vi "Main.vi"() -> ()   [LabVIEW 2020]
uses:
  controls/message cluster.ctl
  <vilib>/Platform/TimedLoop/XDataNode/timing_clust.ctl
  <vilib>/Platform/TimedLoop/XDataNode/nitl_modes.ctl
  <vilib>/Platform/TimedLoop/XDataNode/wakeup.ctl
  <instrlib>/Marlin Instrument Driver/Public/controls/move parameters.ctl
  <instrlib>/Marlin Instrument Driver/Public/controls/axes.ctl
  <instrlib>/Marlin Instrument Driver/Public/controls/heater.ctl
  <vilib>/Utility/config.llb/Read Key (String).vi
  <vilib>/Utility/config.llb/Read Key (Double).vi
  <vilib>/Utility/config.llb/Write Key (String).vi
  <vilib>/Utility/config.llb/Write Key (Double).vi
  <vilib>/platform/TimedLoop/XDataNode/XDataNode.xnode
  <instrlib>/Marlin Instrument Driver/Marlin Instrument Driver.lvlib
  <vilib>/Utility/config.llb/NI_LVConfig.lvlib
  <vilib>/Platform/TimedLoop/XDataNode/XDNodeRunTimeDep.lvlib
panel:
  in  "Tab Control":T1(tab)
  in  "Disable steppers":bool
  in  "Chamber temp":enum16{"0", "40", "50", "60", "70", "80"}(ring) caption="Enum"
  in  "Bed temp":enum16{"0", "50", "60", "80", "100", "120"}(ring) caption="Enum"
  in  "Nozzle temp":T2(ring) caption="Enum"
  in  "Speed":u32=1000 caption="mm/min"
  in  "Distance":enum16{"0.1", "1", "10", "100"}(ring)=enum."10" caption="mm"
  in  "Fan control":u8(slide) caption="%" scale=0.0..255.0
  in  "Extrude":bool
  in  "Retract":bool
  in  "Home all":bool caption="ALL"
  in  "Home Z":bool
  in  "Z-":bool
  in  "Z+":bool
  in  "Home XY":bool
  in  "XY-":bool
  in  "X-":bool
  in  "XY+":bool
  in  "X-Y+":bool
  in  "Y-":bool
  in  "X+Y-":bool
  in  "X+":bool
  in  "Y+":bool
  in  "Monitor data":bool caption="Monitoring slows down communication"
  in  "Update frequency":u32=1000 caption="ms"
  out "Temperature Chart":dbl[][](graph)
  out "Z min":bool
  out "Y min":bool
  out "X min":bool
  out "Gcode array":string[](array[string])
  in  "Stop Gcode":bool
  in  "Pause Gcode":bool
  in  "Test mode":bool
  out "XY Graph":cluster{"X":dbl, "Y":dbl}[](graph)
  in  "Start Gcode":bool
  in  "Gcode file":path caption="Path"
  out "Position sent":dbl caption="Numeric"
  in  "Test mode":bool
  in  "Start torture":bool
  in  "Axle":enum16{"X", "Y", "Z"}(ring) caption="Enum"
  in  "Speed":u32(slide)=3000 caption="%" scale=0.0..9000.0
  in  "Distance":dbl(slide)=100.0 caption="%" scale=0.0..300.0
  out "Initialized":bool
  in  "Initialize":bool
  in  "Delete":bool
  in  "Save":bool
  in  "Z":dbl caption="Numeric"
  in  "Y":dbl caption="Numeric"
  in  "X":dbl caption="Build volume"
  in  "COM port":refnum<visa-resource-name>
  in  "3D printer":string(combo) caption="Combo Box"
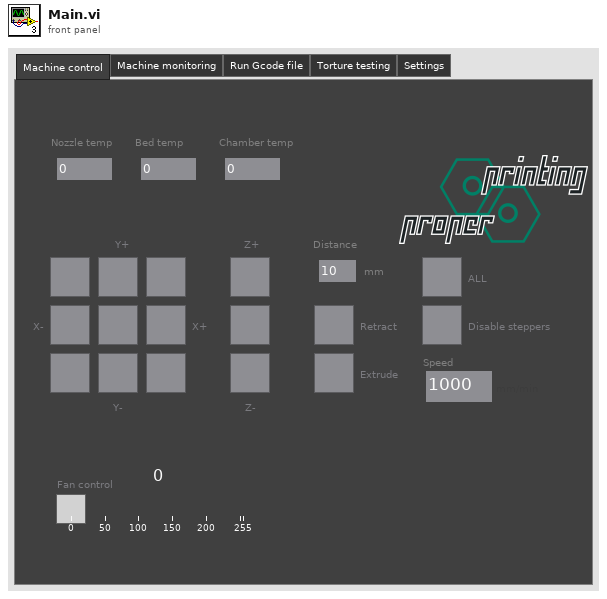
[diagram p1: front panel]
types:
  T1 = enum32{"Machine control", "Machine monitoring", "Run Gcode file", "Torture testing", "Settings"}
  T2 = enum16{"0", "100", "200", "230", "240", "260", "280", "290"}
  T3 = enum8{"Enabled", "Disabled", "Disabled and Grayed Out"}
  T4 = typedef "message cluster.ctl" = cluster{"message":string, "data":variant}
  T5 = typedef "XDNodeRunTimeDep.lvlib/timing_clust.ctl" = cluster{"Expected End [f-1]":u64, "Actual End [f-1]":u64, "Finished Late? [f-1]":bool, "Expected End [i-1]":u64, "Actual End [i-1]":u64, "Finished Late? [i-1]":bool, "Expected Start [i]":u64, "Actual Start [i]":u64, "Expected Start [f]":u64, "Actual Start [f]":u64, "Source Name":string, "Structure Name":string, "Period":i64, "Deadline":i64, "Offset":i64, "Start":i64, "Priority":i32, "Timeout":i32, "Mode":T6, "Wakeup Reason":T7, "Error":errorcluster, "Source Type":string, "Secondary Source Type":string, "Global End Time":u64, "Global Start Time":u64, "Frame Duration":u64, "Iteration Duration":u64, "Assigned CPU":i32, "I/O Scan Engine Mode":u32}
  T6 = typedef "XDNodeRunTimeDep.lvlib/nitl_modes.ctl" = enum32{"No Change", "Process missed periods, maintain original phase", "Discard missed periods, maintain original phase", "Process missed periods, ignore original phase", "Discard missed periods, ignore original phase"}
  T7 = typedef "XDNodeRunTimeDep.lvlib/wakeup.ctl" = enum32{"Normal", "Aborted", "Asynchronous wakeup", "Timing source error", "Timed loop error", "Timeout"}
  T8 = typedef "NI_LVConfig.lvlib/Config Data RefNum.ctl" = refnum<k1>
  T9 = typedef "Marlin Instrument Driver.lvlib/heater.ctl" = enum16{"Hot end", "Bed", "Chamber"}
  T10 = typedef "Marlin Instrument Driver.lvlib/move parameters.ctl" = cluster{"E":dbl, "F":dbl, "X":dbl, "Y":dbl, "Z":dbl}
  T11 = typedef "Marlin Instrument Driver.lvlib/axes.ctl" = cluster{"X":bool, "Y":bool, "Z":bool}
  T12 = typedef "Marlin Instrument Driver.lvlib/end stop status.ctl" = cluster{"x_min":bool, "y_min":bool, "z_min":bool}
  T13 = typedef "Marlin Instrument Driver.lvlib/temperatures.ctl" = cluster{"T":dbl, "T setpoint":dbl, "B":dbl, "B setpoint":dbl}
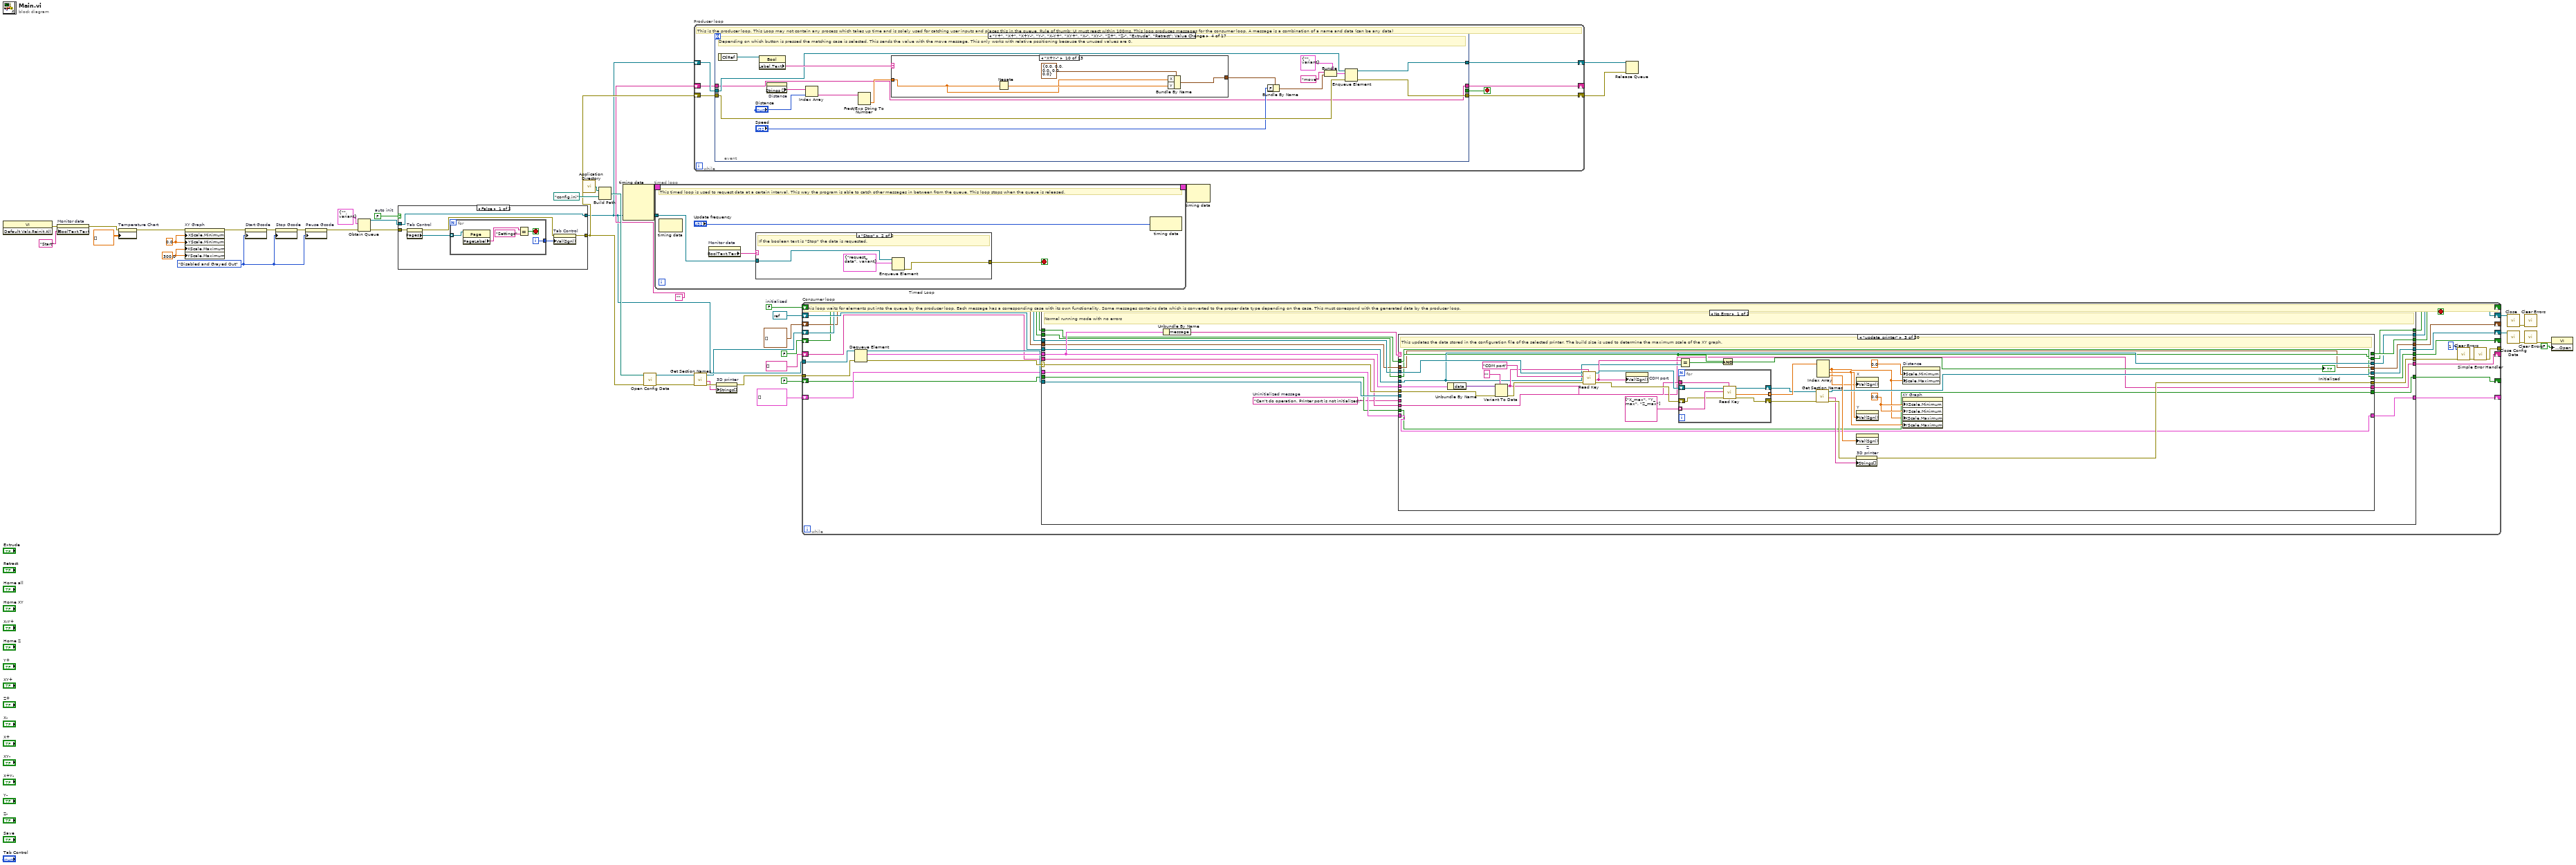
[diagram p0: block diagram]
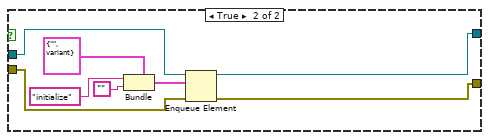
[diagram p2: hidden frame]
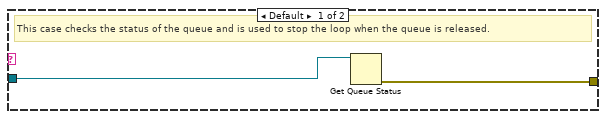
[diagram p3: hidden frame]
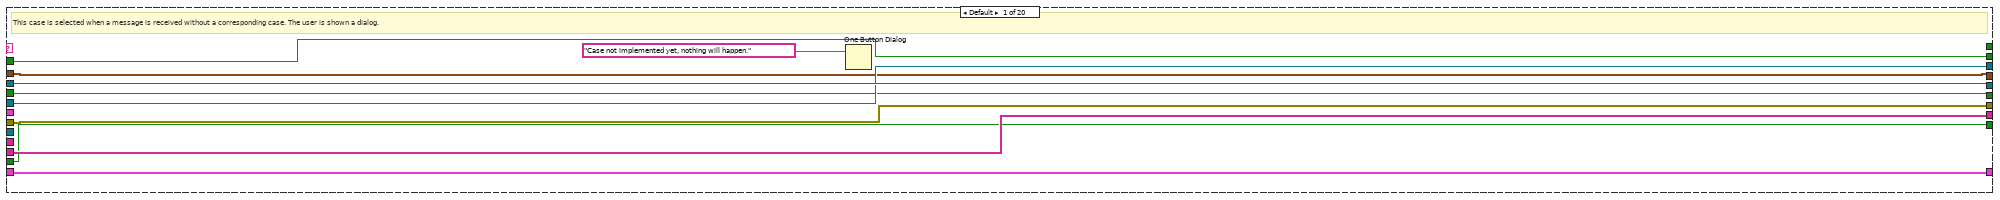
[diagram p4: hidden frame]
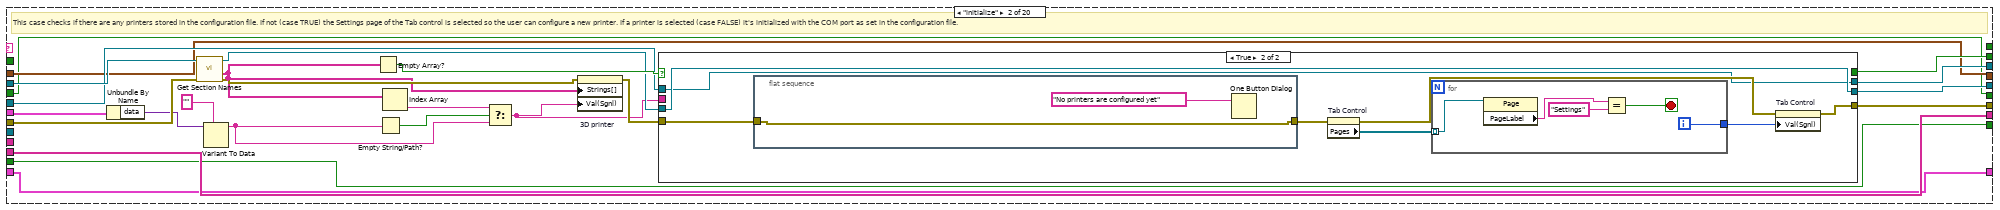
[diagram p5: hidden frame]
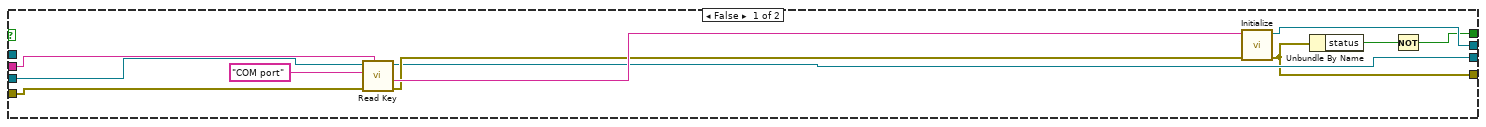
[diagram p6: hidden frame]
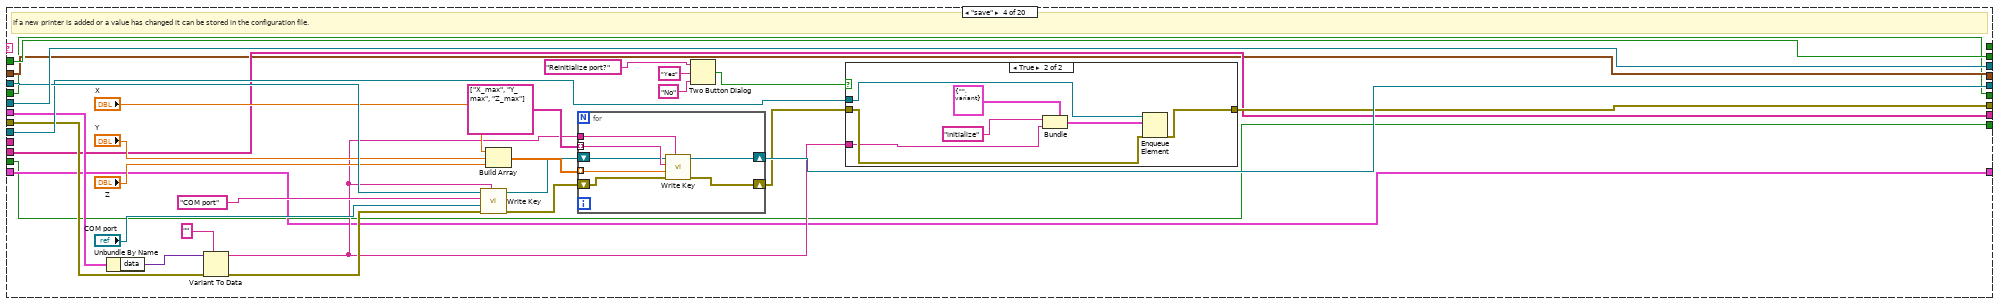
[diagram p7: hidden frame]
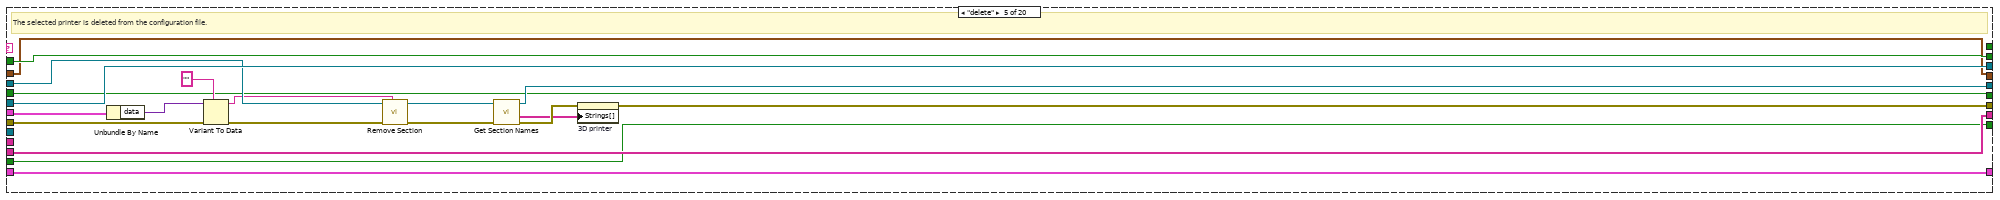
[diagram p9: hidden frame]
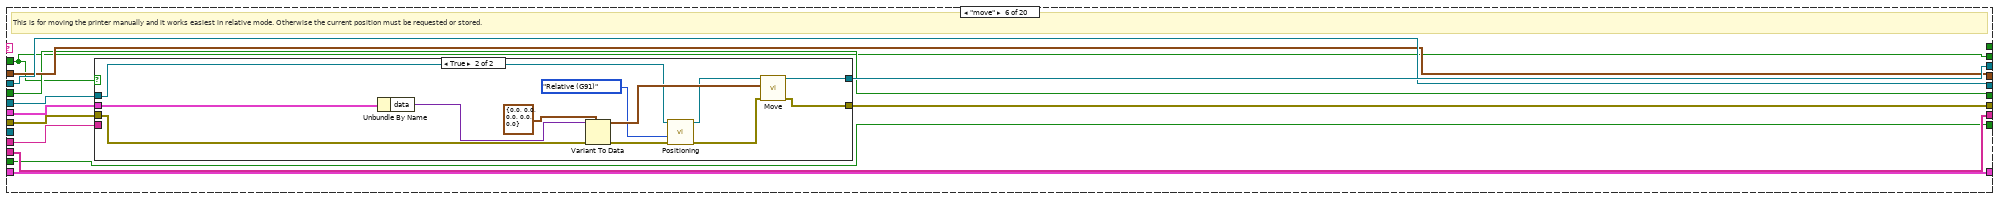
[diagram p10: hidden frame]
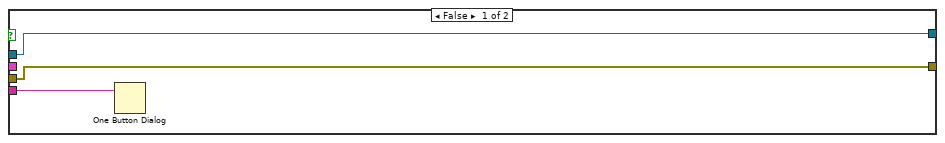
[diagram p11: hidden frame]
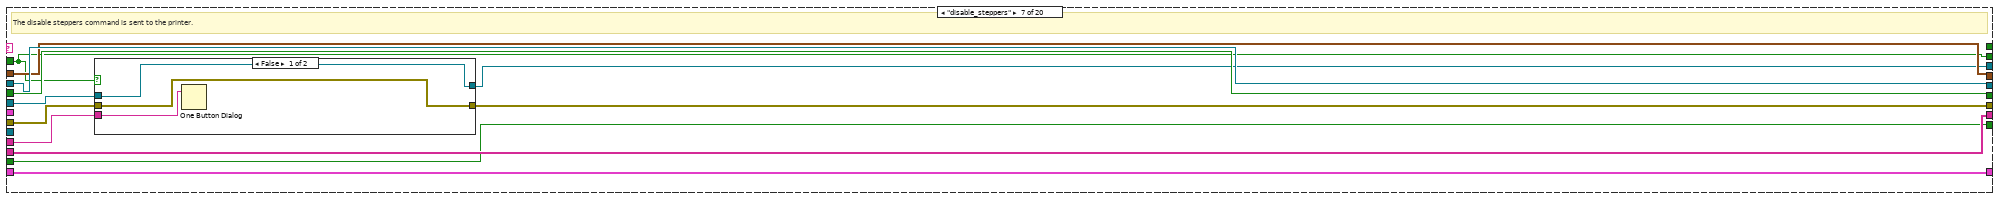
[diagram p12: hidden frame]
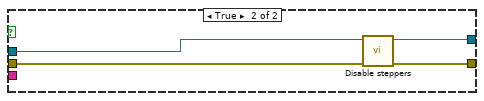
[diagram p13: hidden frame]
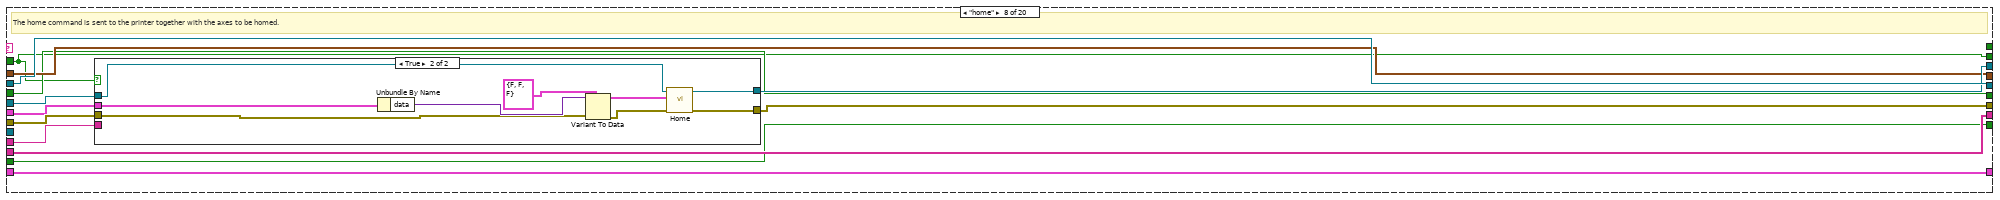
[diagram p14: hidden frame]
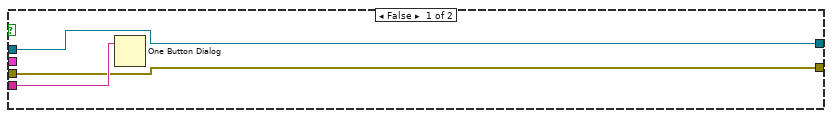
[diagram p15: hidden frame]
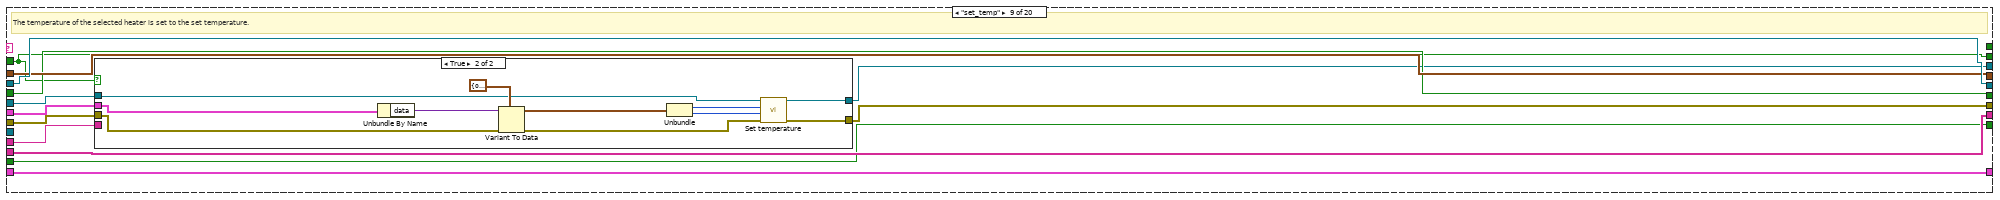
[diagram p16: hidden frame]
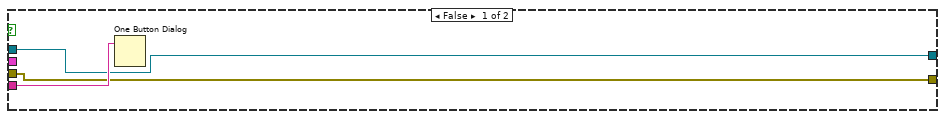
[diagram p17: hidden frame]
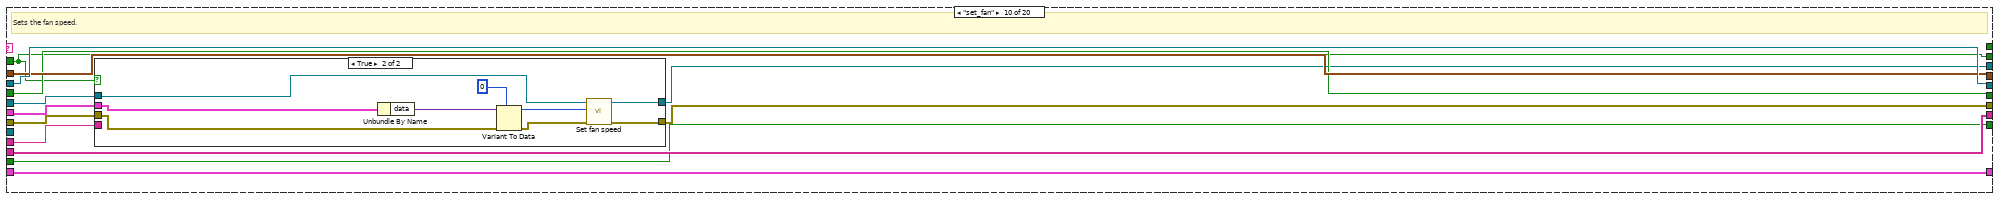
[diagram p18: hidden frame]
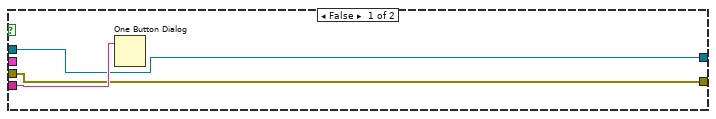
[diagram p19: hidden frame]
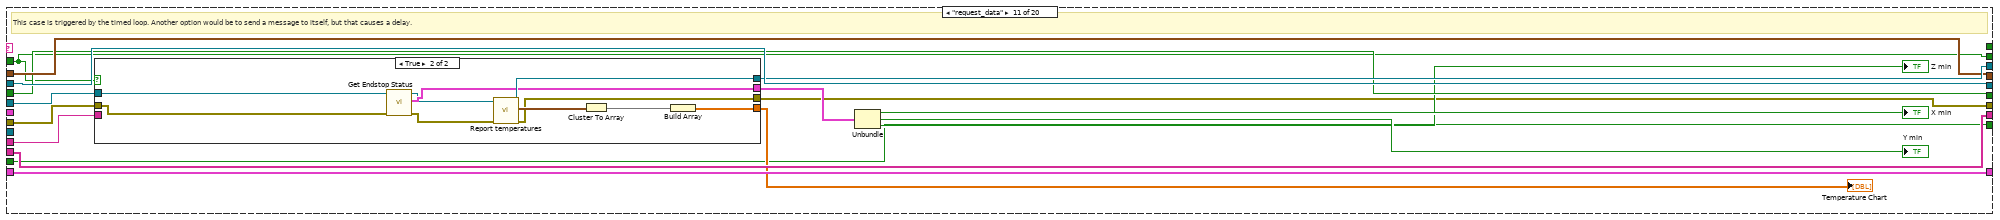
[diagram p20: hidden frame]
diagram:
  w3 = 300.0 ("X Scale.Range:Maximum")
  w4 = 0.0 ("X Scale.Range:Minimum")
  w22 = FALSE  # auto init
  w26 = T3."Disabled and Grayed Out" ("Disabled")
  w40 = FALSE  # initialized
  n1 = invoke class="VI" method="Default Vals.Reinit All"() -> (error out=w10:errorcluster)  [unwired: 3 in, 2 out]
  n2 = property on="Monitor data" class="Bool"(error in=w10, "BoolText.Text"="Start" ("Boolean Text.Text")) -> (error out=w19:errorcluster)  [unwired: 1 in, 1 out]
  n3 = property on="Temperature Chart" class="WFChart (strict)"(error in=w19, "History Data"=dbl[][] []) -> (error out=w2:errorcluster)  [unwired: 1 in, 1 out]
  n4 = property on="XY Graph" class="XYGraph (strict)"(error in=w2, "XScale.Minimum"=w4, "YScale.Minimum"=w4, "XScale.Maximum"=w3, "YScale.Maximum"=w3) -> (error out=w1:errorcluster)  [unwired: 1 in, 1 out]
  n5 = property on="Start Gcode" class="Bool"(error in=w1, "DisabledEnum"=w26) -> (error out=w25:errorcluster)  [unwired: 1 in, 1 out]
  n6 = property on="Stop Gcode" class="Bool"(error in=w25, "DisabledEnum"=w26) -> (error out=w24:errorcluster)  [unwired: 1 in, 1 out]
  n7 = property on="Pause Gcode" class="Bool"(error in=w24, "DisabledEnum"=w26) -> (error out=w11:errorcluster)  [unwired: 1 in, 1 out]
  n8 = Obtain Queue(element data type=T4 {"message"="", "data"=variant}, error in (no error)=w11) -> (queue out=w43:refnum<queue>, error out=w42:errorcluster)  [unwired: 3 in, 1 out]
  n9 = case shown="False" w22 {
    tunnel: w43 -> [w51 w64]
    tunnel: w42 -> [w47 w63]
    tunnel: [w46 w62] -> w36
    tunnel: [w51 w57] -> w27
    frame False {
      n10 = property on="Tab Control" class="TabCtl (strict)"(error in=w47) -> (error out=w48:errorcluster, "Pages"=w49:refnum<vi>[])  [unwired: 1 in, 1 out]
      n11 = for {
        tunnel: w49 -> [w56] mode=indexing
        tunnel: [w52] -> w50
        i -> [w52]
        stop <- w53 stop-if-true
        n12 = property class="Page"(reference=w56) -> ("PageLabel"=w55:string)  [unwired: 1 in, 2 out]
        n13 = Equal?(x=w55, y="Settings") -> (x = y?=w53:bool)
      }
      n14 = property on="Tab Control" class="TabCtl (strict)"(error in=w48, "Val(Sgnl)"=w50) -> (error out=w46:errorcluster)  [unwired: 1 in, 1 out]
    }
    frame True {
      n15 = Bundle(cluster=T4 {"message"="", "data"=variant}, "message"="initialize", "data"="") -> (w58:T4)
      n16 = Enqueue Element(queue=w64, element=w58, error in (no error)=w63) -> (queue out=w57:refnum<queue>, error out=w62:errorcluster)  [unwired: 1 in, 1 out]
    }
  }
  n17 = call <vilib>:"Application Directory.vi"() -> ("Application Directory"=w39:path)
  n18 = Build Path(base path=w39, name or relative path=path "config.ini") -> (appended path=w37:path)
  n19 = node-c288() -> (w29:T5)  [unwired: 4 in]
  n20 = call <vilib>:"Open Config Data.vi"("error in (no error)"=w36, "configuration file path"=w37) -> ("error out"=w17:errorcluster, "refnum"=w16:T8)  [unwired: 7 in, 1 out]
  n21 = timed-loop "Timed Loop" {
    timing: w29 -> [_]
    timing-out: [_] -> w28
    tunnel: w27 -> [w67]
    stop <- w65 stop-if-true
    # "This timed loop is used to request data at a certain interval. This way the program is able to catch other messages in between from the queue. This loop stops when the queue is released."
    n22 = node-c288() -> ()  [unwired: 1 in, 1 out]
    n23 = property on="Monitor data" class="Bool"() -> ("BoolText.Text"=w66:string)  [unwired: 2 in, 2 out]
    n24 = case shown="\"Stop\"" w66 {
      tunnel: w67 -> [w69 w73]
      tunnel: [w70 w72] -> w65
      frame Default {
        # "This case checks the status of the queue and is used to stop the loop when the queue is released."
        n25 = Get Queue Status(queue=w69) -> (error out=w70:errorcluster)  [unwired: 2 in, 7 out]
      }
      frame "Stop" {
        # "If the boolean text is \"Stop\" the data is requested."
        n26 = Enqueue Element(queue=w73, element=T4 {"message"="request_data", "data"=variant}) -> (error out=w72:errorcluster)  [unwired: 2 in, 2 out]
      }
    }
    n27 = node-c288("Update frequency") -> ()  [unwired: 1 out]
  }
  n28 = while "Producer loop" {
    shift-right: [w81] -> w44
    shift-left: w36 -> [w82]
    shift-right: [w80] -> w9
    shift-left: w27 -> [w83]
    shift-right: [w79] -> _
    shift-left: "" -> [w78]
    stop <- w84 stop-if-true
    # "This is the producer loop. This Loop may not contain any process which takes up time and is solely used for catching user inputs and places this in the queue. Rule of thumb: UI must react within 100ms. This loop produces messages for the consumer loop. A message is a combination of a name and data (can be any data)"
    n29 = event shown="[3] \"Y+\", \"X+\", \"X+Y-\", \"Y-\", \"X-Y+\", \"XY+\", \"X-\", \"XY-\", \"Z+\", \"Z-\", \"Extrude\", \"Retract\": Value Change" {
      selector: _ -> [_ _ _ _ _ _ _ _ _ _ _ _ _ _ _ _ _]
      dyn-events: _ -> [_ _ _ _ _ _ _ _ _ _ _ _ _ _ _ _ _]
      timeout: _ -> [_ _ _ _ _ _ _ _ _ _ _ _ _ _ _ _ _]
      tunnel: [_ _ _ _ _ _ _ _ _ _ _ _ _ _ _ _ TRUE] -> w84
      tunnel: w83 -> [w86 w92 w102 w130 w182 w189 w203 w217 w226 w235 w254 w264 w280 w301 w305 w313 w324]
      tunnel: w82 -> [w87 w91 w100 w125 w180 w186 w201 w213 w223 w236 w252 w262 w278 w299 w304 w312 w322]
      tunnel: [w87 w90 w99 w124 w179 w185 w199 w208 w222 w230 w251 w261 w277 w298 w303 w311 w321] -> w81
      tunnel: [w86 w89 w101 w126 w181 w188 w202 w217 w224 w234 w253 w263 w279 w300 w302 w310 w320] -> w80
      tunnel: [w85 w88 w112 w120 w184 w195 w207 w219 w229 w238 w256 w265 w281 w295 w306 w314 w319] -> w79
      tunnel: w78 -> [w85 w88 w112 w120 w184 w195 w207 w219 w229 w238 w256 w265 w281 w295 _ w314 w319]
      event Timeout {
        # "This event will never trigger (timeout = -1)"
        n30 = event-data() -> ()  [unwired: 1 in, 3 out]
      }
      event "Initialize": Value Change {
        # "The initialize message is sent to the consumer loop."
        n31 = event-data() -> ()  [unwired: 1 in, 6 out]
        n32 = Bundle(cluster=T4 {"message"="", "data"=variant}, "message"="initialize", "data"=w88) -> (w93:T4)
        n33 = Enqueue Element(queue=w92, element=w93, error in (no error)=w91) -> (queue out=w89:refnum<queue>, error out=w90:errorcluster)  [unwired: 1 in, 1 out]
      }
      event "Nozzle temp", "Bed temp", "Chamber temp": Value Change {
        # "This event looks at the lable of which input has changed which corresponds with a case. The data is sent together with the set_temp message to the consumer loop."
        n34 = event-data() -> ("CtlRef"=w111:refnum<vi>)  [unwired: 1 in]
        n35 = property class="Enum"(reference=w111) -> ("Label.Text"=w110:string, "Strings []"=w109:string[])  [unwired: 1 in, 2 out]
        n36 = case shown="\"Chamber temp\"" w110 {
          tunnel: ["Bed temp" "Chamber temp" "Nozzle temp"] -> w108
          tunnel: [heater."Bed" ("Heater") heater."Chamber" ("Heater") heater."Hot end" ("Heater")] -> w96
          frame "Bed temp" {
          }
          frame "Chamber temp" {
          }
          frame "Nozzle temp", Default {
          }
        }
        n37 = Index Array(array=w109, index=w108) -> (element=w107:string)
        n38 = Decimal String To Number(string=w107) -> (number=w106:i32)  [unwired: 2 in, 1 out]
        n39 = Bundle(cluster=cluster{"setpoint":i32, "Heater":T9} {"setpoint"=0, "Heater"=enum."Hot end"} ("output cluster"), "setpoint"=w106, "Heater"=w96) -> (w98:cluster{"setpoint":i32, "Heater":T9})
        n40 = Bundle(cluster=T4 {"message"="", "data"=variant}, "message"="set_temp", "data"=w98) -> (w103:T4)
        n41 = Enqueue Element(queue=w102, element=w103, error in (no error)=w100) -> (queue out=w101:refnum<queue>, error out=w99:errorcluster)  [unwired: 1 in, 1 out]
      }
      event "Y+", "X+", "X+Y-", "Y-", "X-Y+", "XY+", "X-", "XY-", "Z+", "Z-", "Extrude", "Retract": Value Change {
        # "Depending on which button is pressed the matching case is selected. This sends the value with the move message. This only works with relative positioning because the unused values are 0."
        n42 = event-data() -> ("CtlRef"=w135:refnum<vi>)  [unwired: 1 in]
        n43 = property class="Bool"(reference=w135) -> ("Label.Text"=w134:string)  [unwired: 1 in, 2 out]
        n44 = property on="Distance" class="Enum (strict)"() -> ("Strings []"=w133:string[])  [unwired: 2 in, 2 out]
        n45 = Index Array(array=w133, index="Distance") -> (element=w132:string)
        n46 = Fract/Exp String To Number(string=w132) -> (number=w131:dbl)  [unwired: 3 in, 1 out]
        n47 = case shown="\"X+Y-\"" w134 {
          tunnel: w131 -> [_ w137 w140 w143 w146 w150 w154 w157 w161 w164 w168 w172 w176]
          tunnel: [_ w136 w139 w142 w147 w151 w155 w158 w162 w166 w170 w173 w177] -> w123
          frame Default {
          }
          frame "X+" {
            n48 = Bundle By Name(cluster=T10 {"E"=0.0, "F"=0.0, "X"=0.0, "Y"=0.0, "Z"=0.0} ("Distances"), "X"=w137) -> (w136:T10)
          }
          frame "Y+" {
            n49 = Bundle By Name(cluster=T10 {"E"=0.0, "F"=0.0, "X"=0.0, "Y"=0.0, "Z"=0.0} ("Distances"), "Y"=w140) -> (w139:T10)
          }
          frame "Z+" {
            n50 = Bundle By Name(cluster=T10 {"E"=0.0, "F"=0.0, "X"=0.0, "Y"=0.0, "Z"=0.0} ("Distances"), "Z"=w143) -> (w142:T10)
          }
          frame "X-" {
            n51 = Negate(x=w146) -> (-x=w145:dbl)
            n52 = Bundle By Name(cluster=T10 {"E"=0.0, "F"=0.0, "X"=0.0, "Y"=0.0, "Z"=0.0} ("Distances"), "X"=w145) -> (w147:T10)
          }
          frame "Y-" {
            n53 = Negate(x=w150) -> (-x=w149:dbl)
            n54 = Bundle By Name(cluster=T10 {"E"=0.0, "F"=0.0, "X"=0.0, "Y"=0.0, "Z"=0.0} ("Distances"), "Y"=w149) -> (w151:T10)
          }
          frame "Z-" {
            n55 = Negate(x=w154) -> (-x=w153:dbl)
            n56 = Bundle By Name(cluster=T10 {"E"=0.0, "F"=0.0, "X"=0.0, "Y"=0.0, "Z"=0.0} ("Distances"), "Z"=w153) -> (w155:T10)
          }
          frame "XY+" {
            n57 = Bundle By Name(cluster=T10 {"E"=0.0, "F"=0.0, "X"=0.0, "Y"=0.0, "Z"=0.0} ("Distances"), "X"=w157, "Y"=w157) -> (w158:T10)
          }
          frame "XY-" {
            n58 = Negate(x=w161) -> (-x=w160:dbl)
            n59 = Bundle By Name(cluster=T10 {"E"=0.0, "F"=0.0, "X"=0.0, "Y"=0.0, "Z"=0.0} ("Distances"), "X"=w160, "Y"=w160) -> (w162:T10)
          }
          frame "X+Y-" {
            n60 = Negate(x=w164) -> (-x=w165:dbl)
            n61 = Bundle By Name(cluster=T10 {"E"=0.0, "F"=0.0, "X"=0.0, "Y"=0.0, "Z"=0.0} ("Distances"), "X"=w164, "Y"=w165) -> (w166:T10)
          }
          frame "X-Y+" {
            n62 = Negate(x=w168) -> (-x=w169:dbl)
            n63 = Bundle By Name(cluster=T10 {"E"=0.0, "F"=0.0, "X"=0.0, "Y"=0.0, "Z"=0.0} ("Distances"), "X"=w169, "Y"=w168) -> (w170:T10)
          }
          frame "Extrude" {
            n64 = Bundle By Name(cluster=T10 {"E"=0.0, "F"=0.0, "X"=0.0, "Y"=0.0, "Z"=0.0} ("Distances"), "E"=w172) -> (w173:T10)
          }
          frame "Retract" {
            n65 = Negate(x=w176) -> (-x=w175:dbl)
            n66 = Bundle By Name(cluster=T10 {"E"=0.0, "F"=0.0, "X"=0.0, "Y"=0.0, "Z"=0.0} ("Distances"), "E"=w175) -> (w177:T10)
          }
        }
        n67 = Bundle By Name(cluster=w123, "F"="Speed") -> (w122:T10)
        n68 = Bundle(cluster=T4 {"message"="", "data"=variant}, "message"="move", "data"=w122) -> (w129:T4)
        n69 = Enqueue Element(queue=w130, element=w129, error in (no error)=w125) -> (queue out=w126:refnum<queue>, error out=w124:errorcluster)  [unwired: 1 in, 1 out]
      }
      event "Disable steppers": Value Change {
        # "The disable_steppers message is sent to the consumer loop."
        n70 = event-data() -> ()  [unwired: 1 in, 6 out]
        n71 = Enqueue Element(queue=w182, element=T4 {"message"="disable_steppers", "data"=variant}, error in (no error)=w180) -> (queue out=w181:refnum<queue>, error out=w179:errorcluster)  [unwired: 1 in, 1 out]
      }
      event "Home XY", "Home Z", "Home all": Value Change {
        # "The home message is sent to the consumer loop together with the data which tells which axes to home."
        n72 = event-data() -> ("CtlRef"=w194:refnum<vi>)  [unwired: 1 in]
        n73 = property class="Bool"(reference=w194) -> ("Label.Text"=w193:string)  [unwired: 1 in, 2 out]
        n74 = case shown="\"Home Z\"" w193 {
          tunnel: [T11 {"X"=TRUE, "Y"=TRUE, "Z"=TRUE} ("Axes") T11 {"X"=TRUE, "Y"=TRUE, "Z"=FALSE} ("Axes") T11 {"X"=FALSE, "Y"=FALSE, "Z"=TRUE} ("Axes")] -> w187
          frame "Home all", Default {
          }
          frame "Home XY" {
          }
          frame "Home Z" {
          }
        }
        n75 = Bundle(cluster=T4 {"message"="", "data"=variant}, "message"="home", "data"=w187) -> (w190:T4)
        n76 = Enqueue Element(queue=w189, element=w190, error in (no error)=w186) -> (queue out=w188:refnum<queue>, error out=w185:errorcluster)  [unwired: 1 in, 1 out]
      }
      event "Fan control": Value Change {
        # "The set_fan message is sent to the consumer loop. The NewVal is used and the event is triggered immediately when the Fan control slider is moved. This slows down communication and should therefore not be performed when a Gcode is running."
        n77 = event-data() -> ("NewVal"=w200:u8)  [unwired: 1 in]
        n78 = Bundle(cluster=T4 {"message"="", "data"=variant}, "message"="set_fan", "data"=w200) -> (w204:T4)
        n79 = Enqueue Element(queue=w203, element=w204, error in (no error)=w201) -> (queue out=w202:refnum<queue>, error out=w199:errorcluster)  [unwired: 1 in, 1 out]
      }
      event "Monitor data": Value Change {
        w211 = "Start" ("y")
        # "This event changes the boolean text of the Monitor data button from Start to Stop and vice versa. This is used to enable or disable the timed loop data request."
        n80 = event-data() -> ("CtlRef"=w218:refnum<vi>)  [unwired: 1 in, 2 out]
        n81 = property class="Bool"(reference=w218, error in=w213) -> (reference out=w215:refnum<vi>, error out=w214:errorcluster, "BoolText.Text"=w216:string)
        n82 = Equal?(x=w216, y=w211) -> (x = y?=w212:bool)
        n83 = Select(t="Stop", s=w212, f=w211) -> (s? t:f=w209:string)
        n84 = property class="Bool"(reference=w215, error in=w214, "BoolText.Text"=w209) -> (error out=w208:errorcluster)  [unwired: 1 out]
      }
      event "Gcode file": Value Change {
        # "The load_gcode message is sent to the consumer loop together with the selected path."
        n85 = event-data() -> ("NewVal"=w221:path)  [unwired: 1 in]
        n86 = Strip Path(path=w221) -> (name=w220:string)  [unwired: 1 out]
        n87 = property on="Gcode file" class="Path"("Text.Text"=w220) -> ()  [unwired: 2 in, 2 out]
        n88 = Bundle(cluster=T4 {"message"="", "data"=variant} ("element"), "message"="load_gcode", "data"=w221) -> (w225:T4)
        n89 = Enqueue Element(queue=w226, element=w225, error in (no error)=w223) -> (queue out=w224:refnum<queue>, error out=w222:errorcluster)  [unwired: 1 in, 1 out]
      }
      event "Start Gcode": Value Change {
        # "The run_gcode message is sent to the consumer loop after the user confirms the message. The current index of the Gcode array (first array element is 0) is sent as data."
        n90 = event-data() -> ()  [unwired: 1 in, 4 out]
        n91 = Two Button Dialog(message="Run selected program?", 1:"No" ("F button name (\"Cancel\")"), 2:"Yes" ("T button name (\"OK\")")) -> (T button?=w233:bool)
        n92 = case shown="True" w233 {
          tunnel: w236 -> [w239 w247]
          tunnel: w235 -> [w240 w246]
          tunnel: [w240 w245] -> w234
          tunnel: [w239 w243] -> w230
          frame False {
          }
          frame True {
            w241 = T3."Enabled" ("Disabled")
            n93 = property on="Stop Gcode" class="Bool"("DisabledEnum"=w241) -> ()  [unwired: 2 in, 2 out]
            n94 = property on="Pause Gcode" class="Bool"("DisabledEnum"=w241) -> ()  [unwired: 2 in, 2 out]
            n95 = Bundle(cluster=T4 {"message"="", "data"=variant} ("element"), "message"="run_gcode", "data"=0) -> (w248:T4)
            n96 = property on="Start Gcode" class="Bool"("DisabledEnum"=T3."Disabled and Grayed Out" ("Disabled")) -> ()  [unwired: 2 in, 2 out]
            n97 = Enqueue Element(queue=w246, element=w248, error in (no error)=w247) -> (queue out=w245:refnum<queue>, error out=w243:errorcluster)  [unwired: 1 in, 1 out]
          }
        }
      }
      event "Pause Gcode": Value Change {
        # "The pause_gcode message is sent to the consumer loop."
        n98 = event-data() -> ()  [unwired: 1 in, 1 out]
        n99 = Enqueue Element(queue=w254, element=T4 {"message"="pause_gcode", "data"=variant}, error in (no error)=w252) -> (queue out=w253:refnum<queue>, error out=w251:errorcluster)  [unwired: 1 in, 1 out]
      }
      event "Stop Gcode": Value Change {
        # "The stop_gcode message is sent to the consumer loop after the user confirms the message."
        n100 = event-data() -> ()  [unwired: 1 in, 1 out]
        n101 = Two Button Dialog(message="Stop current running program?", 1:"No" ("F button name (\"Cancel\")"), 2:"Yes" ("T button name (\"OK\")")) -> (T button?=w257:bool)
        n102 = case shown="True" w257 {
          tunnel: w264 -> [w267 w271]
          tunnel: [w267 w270] -> w263
          tunnel: w262 -> [w266 w269]
          tunnel: [w266 w268] -> w261
          frame False {
          }
          frame True {
            n103 = Enqueue Element At Opposite End(queue=w271, element=T4 {"message"="stop_gcode", "data"=variant}, error in (no error)=w269) -> (queue out=w270:refnum<queue>, error out=w268:errorcluster)  [unwired: 1 in, 1 out]
          }
        }
      }
      event "Start torture": Value Change {
        # "Depending on the boolean text the start_torture or stop_torture  message is sent to the consumer loop. The boolean text is changed from start to stop and vice versa when pressed."
        n104 = event-data() -> ("CtlRef"=w276:refnum<vi>)  [unwired: 1 in, 5 out]
        n105 = property class="Bool"(reference=w276) -> (reference out=w274:refnum<vi>, "BoolText.Text"=w275:string)  [unwired: 1 in, 1 out]
        n106 = case shown="\"Start\"" w275 {
          tunnel: w280 -> [w286 w292]
          tunnel: [w285 w291] -> w279
          tunnel: w278 -> [w284 w290]
          tunnel: [w283 w289] -> w277
          tunnel: ["Stop" "Start"] -> w273
          frame "Start" {
            n107 = Enqueue Element(queue=w286, element=T4 {"message"="start_torture", "data"=variant}, error in (no error)=w284) -> (queue out=w285:refnum<queue>, error out=w283:errorcluster)  [unwired: 1 in, 1 out]
          }
          frame "Stop", Default {
            n108 = Enqueue Element At Opposite End(queue=w292, element=T4 {"message"="stop_torture", "data"=variant}, error in (no error)=w290) -> (queue out=w291:refnum<queue>, error out=w289:errorcluster)  [unwired: 1 in, 1 out]
          }
        }
        n109 = property class="Bool"(reference=w274, "BoolText.Text"=w273) -> ()  [unwired: 1 in, 2 out]
      }
      event "Save": Value Change {
        # "The save message is sent to the consumer loop."
        n110 = event-data() -> ()  [unwired: 1 in, 6 out]
        n111 = Bundle(cluster=T4 {"message"="", "data"=variant}, "message"="save", "data"=w295) -> (w294:T4)
        n112 = Enqueue Element(queue=w301, element=w294, error in (no error)=w299) -> (queue out=w300:refnum<queue>, error out=w298:errorcluster)  [unwired: 1 in, 1 out]
      }
      event "3D printer": Value Change {
        # "The update_printer message is sent to the consumer loop."
        n113 = event-data() -> ("NewVal"=w306:string)  [unwired: 1 in]
        n114 = Bundle(cluster=T4 {"message"="", "data"=variant}, "message"="update_printer", "data"=w306) -> (w307:T4)
        n115 = Enqueue Element(queue=w305, element=w307, error in (no error)=w304) -> (queue out=w302:refnum<queue>, error out=w303:errorcluster)  [unwired: 1 in, 1 out]
      }
      event "Delete": Value Change {
        # "The delete message is sent to the consumer loop."
        n116 = event-data() -> ()  [unwired: 1 in, 1 out]
        n117 = Bundle(cluster=T4 {"message"="", "data"=variant}, "message"="delete", "data"=w314) -> (w315:T4)
        n118 = Enqueue Element(queue=w313, element=w315, error in (no error)=w312) -> (queue out=w310:refnum<queue>, error out=w311:errorcluster)  [unwired: 1 in, 1 out]
      }
      event Panel Close? {
        # "The close message is sent to the consumer loop when the front panel is closed by the user. The message is discarded so the program can close the port first. The program quits after all loops are stopped."
        n119 = event-data() -> ()  [unwired: 1 in, 4 out]
        n120 = Enqueue Element At Opposite End(queue=w324, element=T4 {"message"="close", "data"=variant}, error in (no error)=w322) -> (queue out=w320:refnum<queue>, error out=w321:errorcluster)  [unwired: 1 in, 1 out]
        n121 = event-data("Discard?"=TRUE) -> ()  [unwired: 1 in, 1 out]
      }
    }
  }
  n122 = call <vilib>:"Get Section Names.vi"("error in (no error)"=w17, "refnum"=w16) -> ("error out"=w13:errorcluster, "section names"=w12:string[], "refnum out"=w15:T8)  [unwired: 7 in]
  n123 = property on="3D printer" class="CmbBox"(error in=w13, "Strings[]"=w12) -> (error out=w14:errorcluster)  [unwired: 1 in, 1 out]
  n124 = while "Consumer loop" {
    tunnel: w27 -> [w351]
    shift-right: [w346] -> w8
    shift-left: refnum<visa-resource-name> refnum ("VISA resource name out") -> [w344]
    shift-right: [w345] -> w35
    shift-left: w15 -> [w343]
    shift-right: [w342] -> _
    shift-left: w40 -> [w341]
    shift-right: [w339] -> _
    shift-left: string[] [] ("Gcode Array") -> [w338]
    shift-right: [w336] -> _
    shift-left: cluster{"X":dbl, "Y":dbl}[] [] ("XY Graph 2") -> [w337]
    shift-right: [w331] -> _
    shift-left: FALSE -> [w332]
    shift-right: [w330] -> _
    shift-left: T4[] [] ("remaining elements") -> [w329]
    tunnel: w14 -> [w347]
    tunnel: [w328] -> _
    shift-right: [w326] -> _
    shift-left: FALSE -> [w327]
    stop <- w349 stop-if-true
    # "This loop waits for elements put into the queue by the producer loop. Each message has a corresponding case with its own functionality. Some messages contains data which is converted to the proper data type depending on the case. This must correspond with the generated data by the producer loop."
    n125 = Dequeue Element(queue=w351, error in (no error)=w347) -> (queue out=w340:refnum<queue>, element=w350:T4, error out=w348:errorcluster)  [unwired: 1 in, 1 out]
    n126 = case shown="No Error" w348 {
      selector: w348 -> [w371 _]
      tunnel: w350 -> [w373 _]
      tunnel: [w372 TRUE] -> w349
      tunnel: [w370 w985] -> w346
      tunnel: [w369 w984] -> w345
      tunnel: w344 -> [w368 w985]
      tunnel: w343 -> [w367 w984]
      tunnel: [w366 _] -> w342
      tunnel: w341 -> [w365 _]
      tunnel: w340 -> [w364 _]
      tunnel: [w363 _] -> w335
      tunnel: [w362 w982] -> w339
      tunnel: w338 -> [w361 w982]
      tunnel: w337 -> [w360 w981]
      tunnel: [w359 w981] -> w336
      tunnel: w332 -> [w358 w980]
      tunnel: [w357 w980] -> w331
      tunnel: [w356 w979] -> w330
      tunnel: w329 -> [w355 w979]
      tunnel: w327 -> [w354 w978]
      tunnel: [w353 w978] -> w326
      frame No Error {
        w352 = "Can't do operation. Printer port is not initialized."  # Uninitialized message
        # "Normal running mode with no errors"
        n127 = Unbundle By Name(w373) -> ("message"=w374:string)
        n128 = case shown="\"update_printer\"" w374 {
          tunnel: w373 -> [_ w397 w465 w489 w532 w553 _ w597 w620 w647 _ w707 w756 _ _ _ _ _ _ _]
          tunnel: [_ _ _ _ _ _ _ _ _ _ _ _ _ _ _ _ _ _ _ TRUE] -> w372
          tunnel: [w384 w405 w449 w490 w526 w552 w573 w595 w617 w644 w667 w702 w748 w771 w815 w834 w840 w913 w957 w968] -> w363
          tunnel: w371 -> [w384 w402 w464 w486 w535 w551 w574 w598 w616 w643 w669 w706 w755 w772 w816 w834 w844 w918 w958 w968]
          tunnel: [w382 w406 w447 w505 w540 w550 w572 w596 w618 w645 w679 w709 w751 w768 w821 w833 w839 w916 w967 w969] -> w370
          tunnel: [w383 w404 w451 w493 w527 w549 w580 w600 w625 w652 w681 w708 w759 w781 w820 w832 w850 w926 w966 w976] -> w369
          tunnel: w368 -> [w382 w400 w447 w505 w540 w548 w575 w599 w619 w646 w680 w709 w753 w769 w821 w833 w845 w917 w967 w969]
          tunnel: w367 -> [w383 w401 w462 w503 w538 w549 w580 w600 w625 w652 w681 w708 w759 w781 w820 w832 w850 w926 w966 w976]
          tunnel: [w381 w403 w446 w504 w539 w542 w569 w589 w614 w640 w665 w698 w758 w780 w819 w831 w836 w925 w965 w975] -> w366
          tunnel: w365 -> [w381 _ w446 w504 w539 w542 w569 w589 w614 w640 w665 w698 w758 w780 w819 w831 w836 w925 w965 w975]
          tunnel: w364 -> [_ _ _ w492 _ _ _ _ _ _ _ _ w747 w776 w817 _ w841 w912 w959 _]
          tunnel: [w380 w389 w443 w479 w525 w547 w579 w594 w624 w651 w678 w700 w746 w779 _ w830 w849 w924 w964 w974] -> w362
          tunnel: w361 -> [w380 w389 w443 w479 w525 w547 w579 w594 w624 w651 w678 _ w746 w779 _ w830 w849 w924 w964 w974]
          tunnel: w360 -> [w379 w388 w442 w478 w524 w546 w578 w593 w623 w650 w677 w705 w739 w778 w818 w828 w848 w923 w963 w973]
          tunnel: [w379 w388 w442 w478 w524 w546 w578 w593 w623 w650 w677 w705 w737 w778 w818 w828 w848 w923 w963 w973] -> w359
          tunnel: w358 -> [w378 w387 w439 w477 w523 w545 w577 w592 w622 w649 w676 w704 w730 w777 w814 w827 w847 w922 w962 w972]
          tunnel: [w378 w387 w439 w477 w523 w545 w577 w592 w622 w649 w676 w704 w730 w775 w814 w827 w847 w922 w962 w972] -> w357
          tunnel: [w377 w386 w438 w476 w522 w544 w576 w591 w621 w648 w675 w703 w729 w774 _ w826 w846 w921 w961 w971] -> w356
          tunnel: w355 -> [w377 w386 w438 w476 w522 w544 w576 w591 w621 w648 w675 w703 w729 w773 _ w826 w846 w921 w961 w971]
          tunnel: w354 -> [w376 w385 w437 w475 w521 w543 w571 w590 w615 w642 w668 w701 w728 w770 w812 w824 _ w906 w960 w970]
          tunnel: [w376 w385 w437 w475 w521 w543 w571 w590 w615 w642 w668 w701 w728 w770 w812 w824 FALSE w905 w960 w970] -> w353
          tunnel: w352 -> [_ _ _ _ _ w541 w570 w588 w613 w641 w666 w699 _ _ _ _ w835 _ _ _]
          frame Default {
            # "This case is selected when a message is received without a corresponding case. The user is shown a dialog."
            n129 = One Button Dialog(message="Case not implemented yet, nothing will happen.") -> ()  [unwired: 1 in, 1 out]
          }
          frame "initialize" {
            # "This case checks if there are any printers stored in the configuration file. If not (case TRUE) the Settings page of the Tab control is selected so the user can configure a new printer. If a printer is selected (case FALSE) it's initialized with the COM port as set in the configuration file."
            n130 = Unbundle By Name(w397) -> ("data"=w399:variant)
            n131 = call <vilib>:"Get Section Names.vi"("error in (no error)"=w402, "refnum"=w401) -> ("error out"=w394:errorcluster, "section names"=w392:string[], "refnum out"=w407:T8)  [unwired: 7 in]
            n132 = Variant To Data(type="", Variant=w399) -> (data=w395:string)  [unwired: 1 in, 1 out]
            n133 = Empty Array?(array=w392) -> (empty?=w408:bool)
            n134 = Empty String/Path?(string/path=w395) -> (empty?=w396:bool)
            n135 = Index Array(array=w392) -> (element=w391:string)  [unwired: 1 in]
            n136 = Select(t=w391, s=w396, f=w395) -> (s? t:f=w390:string)
            n137 = property on="3D printer" class="CmbBox"(error in=w394, "Strings[]"=w392, "Val(Sgnl)"=w390) -> (error out=w393:errorcluster)  [unwired: 1 in, 1 out]
            n138 = case shown="True" w408 {
              tunnel: w407 -> [w419 w427]
              tunnel: [w416 w422] -> w406
              tunnel: [w412 w423] -> w405
              tunnel: w393 -> [w414 w425]
              tunnel: [w413 w427] -> w404
              tunnel: [w410 _] -> w403
              tunnel: w400 -> [_ w422]
              tunnel: w390 -> [w409 _]
              frame False {
                n139 = call-poly <vilib>:"Read Key.vi"("section"=w409, "error in (no error)"=w414, "key"="COM port", "refnum"=w419) -> ("error out"=w415:errorcluster, "value"=w417:string, "refnum out"=w413:T8)  [unwired: 4 in, 1 out]
                n140 = call <instrlib>:"Initialize.vi"("error in (no error)"=w415, "VISA resource name"=w417) -> ("error out"=w412:errorcluster, "VISA resource name out"=w416:refnum<visa-resource-name>)  [unwired: 8 in]
                n141 = Unbundle By Name(w412) -> ("status"=w411:bool)
                n142 = Not(x=w411) -> (.not. x?=w410:bool)
              }
              frame True {
                n143 = flat-sequence {
                  tunnel: [w433] -> w426
                  tunnel: w425 -> [w433]
                  frame #0 {
                    n144 = One Button Dialog(message="No printers are configured yet") -> ()  [unwired: 1 in, 1 out]
                  }
                }
                n145 = property on="Tab Control" class="TabCtl (strict)"(error in=w426) -> (error out=w424:errorcluster, "Pages"=w421:refnum<vi>[])  [unwired: 1 in, 1 out]
                n146 = for {
                  tunnel: w421 -> [w432] mode=indexing
                  tunnel: [w428] -> w420
                  i -> [w428]
                  stop <- w429 stop-if-true
                  n147 = property class="Page"(reference=w432) -> ("PageLabel"=w431:string)  [unwired: 1 in, 2 out]
                  n148 = Equal?(x=w431, y="Settings") -> (x = y?=w429:bool)
                }
                n149 = property on="Tab Control" class="TabCtl (strict)"(error in=w424, "Val(Sgnl)"=w420) -> (error out=w423:errorcluster)  [unwired: 1 in, 1 out]
              }
            }
          }
          frame "update_printer" {
            w441 = 0.0 ("X Scale.Range:Minimum")
            # "This updates the data stored in the configuration file of the selected printer. The build size is used to determine the maximum scale of the XY graph."
            n150 = Unbundle By Name(w465) -> ("data"=w467:variant)
            n151 = Variant To Data(error in=w464, type="", Variant=w467) -> (data=w455:string, error out=w463:errorcluster)
            n152 = call-poly <vilib>:"Read Key.vi"("section"=w455, "error in (no error)"=w463, "key"="COM port", "refnum"=w462) -> ("error out"=w456:errorcluster, "value"=w448:string, "refnum out"=w457:T8)  [unwired: 4 in, 1 out]
            n153 = property on="COM port" class="VISAName"("Val(Sgnl)"=w448) -> ()  [unwired: 2 in, 2 out]
            n154 = for {
              tunnel: string[] ["X_max", "Y_max", "Z_max"] -> [w474] mode=indexing
              shift-right: [w471] -> w450
              shift-left: w456 -> [w472]
              shift-right: [w470] -> w452
              shift-left: w457 -> [w473]
              tunnel: [w469] -> w460 mode=indexing
              tunnel: w455 -> [w468]
              n155 = call-poly <vilib>:"Read Key.vi"("section"=w468, "error in (no error)"=w472, "key"=w474, "refnum"=w473) -> ("error out"=w471:errorcluster, "value"=w469:dbl, "refnum out"=w470:T8)  [unwired: 4 in, 1 out]
            }
            n156 = Equal?(x=w448, y=w447) -> (x = y?=w445:bool)
            n157 = And(x=w446, y=w445) -> (x .and. y?=→"Initialized":bool)
            n158 = call <vilib>:"Get Section Names.vi"("error in (no error)"=w450, "refnum"=w452) -> ("error out"=w454:errorcluster, "section names"=w453:string[], "refnum out"=w451:T8)  [unwired: 7 in]
            n159 = Index Array(array=w460) -> (element #1=w436:dbl, element #2=w440:dbl, element #3=w459:dbl)  [unwired: 3 in]
            n160 = property on="X" class="DigNum (strict)"("Val(Sgnl)"=w436) -> ()  [unwired: 2 in, 2 out]
            n161 = property on="Y" class="DigNum (strict)"("Val(Sgnl)"=w440) -> ()  [unwired: 2 in, 2 out]
            n162 = property on="Z" class="DigNum (strict)"("Val(Sgnl)"=w459) -> ()  [unwired: 2 in, 2 out]
            n163 = property on="3D printer" class="CmbBox"(error in=w454, "Strings[]"=w453) -> (error out=w449:errorcluster)  [unwired: 1 in, 1 out]
            n164 = property on="Distance" class="Slide (strict)"("Scale.Minimum"=0.0 ("Scale.Range:Minimum"), "Scale.Maximum"=w436) -> ()  [unwired: 2 in, 2 out]
            n165 = property on="XY Graph" class="XYGraph (strict)"("XScale.Minimum"=w441, "YScale.Minimum"=w441, "XScale.Maximum"=w436, "YScale.Maximum"=w440) -> ()  [unwired: 2 in, 2 out]
          }
          frame "save" {
            # "If a new printer is added or a value has changed it can be stored in the configuration file."
            n166 = Unbundle By Name(w489) -> ("data"=w488:variant)
            n167 = Variant To Data(error in=w486, type="", Variant=w488) -> (data=w484:string, error out=w485:errorcluster)
            n168 = call-poly <vilib>:"Write Key.vi"("section"=w484, "error in (no error)"=w485, "value"="COM port", "key"="COM port", "refnum"=w503) -> ("error out"=w494:errorcluster, "refnum out"=w495:T8)  [unwired: 4 in, 1 out]
            n169 = Build Array("X", "Y", "Z") -> (w497:dbl[])
            n170 = for {
              tunnel: w497 -> [w520] mode=indexing
              tunnel: string[] ["X_max", "Y_max", "Z_max"] -> [w519] mode=indexing
              shift-right: [w516] -> w491
              shift-left: w494 -> [w517]
              shift-right: [w515] -> w493
              shift-left: w495 -> [w518]
              tunnel: w484 -> [w514]
              n171 = call-poly <vilib>:"Write Key.vi"("section"=w514, "error in (no error)"=w517, "value"=w520, "key"=w519, "refnum"=w518) -> ("error out"=w516:errorcluster, "refnum out"=w515:T8)  [unwired: 4 in, 1 out]
            }
            n172 = Two Button Dialog(message="Reinitialize port?", 1:"No" ("F button name (\"Cancel\")"), 2:"Yes" ("T button name (\"OK\")")) -> (T button?=w480:bool)
            n173 = case shown="True" w480 {
              tunnel: w492 -> [_ w513]
              tunnel: w491 -> [w506 w512]
              tunnel: [w506 w511] -> w490
              tunnel: w484 -> [_ w507]
              frame False {
              }
              frame True {
                n174 = Bundle(cluster=T4 {"message"="", "data"=variant}, "message"="initialize", "data"=w507) -> (w508:T4)
                n175 = Enqueue Element(queue=w513, element=w508, error in (no error)=w512) -> (error out=w511:errorcluster)  [unwired: 1 in, 2 out]
              }
            }
          }
          frame "delete" {
            # "The selected printer is deleted from the configuration file."
            n176 = Unbundle By Name(w532) -> ("data"=w537:variant)
            n177 = Variant To Data(error in=w535, type="", Variant=w537) -> (data=w533:string, error out=w534:errorcluster)
            n178 = call <vilib>:"Remove Section.vi"("section"=w533, "error in (no error)"=w534, "refnum"=w538) -> ("error out"=w528:errorcluster, "refnum out"=w529:T8)  [unwired: 6 in, 1 out]
            n179 = call <vilib>:"Get Section Names.vi"("error in (no error)"=w528, "refnum"=w529) -> ("error out"=w531:errorcluster, "section names"=w530:string[], "refnum out"=w527:T8)  [unwired: 7 in]
            n180 = property on="3D printer" class="CmbBox"(error in=w531, "Strings[]"=w530) -> (error out=w526:errorcluster)  [unwired: 1 in, 1 out]
          }
          frame "move" {
            # "This is for moving the printer manually and it works easiest in relative mode. Otherwise the current position must be requested or stored."
            n181 = case shown="True" w542 {
              tunnel: w553 -> [_ w568]
              tunnel: [w556 w564] -> w552
              tunnel: w551 -> [w556 w563]
              tunnel: [w555 w562] -> w550
              tunnel: w548 -> [w555 w559]
              tunnel: w541 -> [w554 _]
              frame False {
                n182 = One Button Dialog(message=w554) -> ()  [unwired: 1 in, 1 out]
              }
              frame True {
                n183 = Unbundle By Name(w568) -> ("data"=w567:variant)
                n184 = Variant To Data(error in=w563, type=T10 {"E"=0.0, "F"=0.0, "X"=0.0, "Y"=0.0, "Z"=0.0} ("Distances"), Variant=w567) -> (data=w565:T10, error out=w561:errorcluster)
                n185 = call <instrlib>:"Positioning.vi"("error in (no error)"=w561, "type"=enum16{"Absolute (G90)", "Relative (G91)"}."Relative (G91)", "VISA resource name"=w559) -> ("error out"=w560:errorcluster, "VISA resource name out"=w558:refnum<visa-resource-name>)  [unwired: 7 in]
                n186 = call <instrlib>:"Move.vi"("error in (no error)"=w560, "Distances"=w565, "VISA resource name"=w558) -> ("error out"=w564:errorcluster, "VISA resource name out"=w562:refnum<visa-resource-name>)  [unwired: 7 in]
              }
            }
          }
          frame "disable_steppers" {
            # "The disable steppers command is sent to the printer."
            n187 = case shown="False" w569 {
              tunnel: w575 -> [w583 w587]
              tunnel: w574 -> [w582 w586]
              tunnel: [w582 w585] -> w573
              tunnel: [w583 w584] -> w572
              tunnel: w570 -> [w581 _]
              frame False {
                n188 = One Button Dialog(message=w581) -> ()  [unwired: 1 in, 1 out]
              }
              frame True {
                n189 = call <instrlib>:"Disable steppers.vi"("error in (no error)"=w586, "VISA resource name"=w587) -> ("error out"=w585:errorcluster, "VISA resource name out"=w584:refnum<visa-resource-name>)  [unwired: 8 in]
              }
            }
          }
          frame "home" {
            # "The home command is sent to the printer together with the axes to be homed."
            n190 = case shown="True" w589 {
              tunnel: w599 -> [w602 w612]
              tunnel: w598 -> [w601 w610]
              tunnel: w597 -> [_ w609]
              tunnel: [w602 w605] -> w596
              tunnel: [w601 w604] -> w595
              tunnel: w588 -> [w603 _]
              frame False {
                n191 = One Button Dialog(message=w603) -> ()  [unwired: 1 in, 1 out]
              }
              frame True {
                n192 = Unbundle By Name(w609) -> ("data"=w611:variant)
                n193 = Variant To Data(error in=w610, type=T11 {"X"=FALSE, "Y"=FALSE, "Z"=FALSE} ("Axes"), Variant=w611) -> (data=w607:T11, error out=w606:errorcluster)
                n194 = call <instrlib>:"Home.vi"("error in (no error)"=w606, "Axes"=w607, "VISA resource name"=w612) -> ("error out"=w604:errorcluster, "VISA resource name out"=w605:refnum<visa-resource-name>)  [unwired: 7 in]
              }
            }
          }
          frame "set_temp" {
            # "The temperature of the selected heater is set to the set temperature."
            n195 = case shown="True" w614 {
              tunnel: w620 -> [_ w639]
              tunnel: w619 -> [w626 w633]
              tunnel: [w626 w632] -> w618
              tunnel: [w627 w631] -> w617
              tunnel: w616 -> [w627 w630]
              tunnel: w613 -> [w628 _]
              frame False {
                n196 = One Button Dialog(message=w628) -> ()  [unwired: 1 in, 1 out]
              }
              frame True {
                n197 = Unbundle By Name(w639) -> ("data"=w638:variant)
                n198 = Variant To Data(error in=w630, type=cluster{"setpoint":i32, "Heater":T9} {"setpoint"=0, "Heater"=enum."Hot end"} ("output cluster"), Variant=w638) -> (data=w636:cluster{"setpoint":i32, "Heater":T9}, error out=w629:errorcluster)
                n199 = Unbundle(w636) -> ("setpoint"=w635:i32, "Heater"=w634:T9)
                n200 = call <instrlib>:"Set temperature.vi"("error in (no error)"=w629, "Heater"=w634, "Temperature"=w635, "VISA resource name"=w633) -> ("error out"=w631:errorcluster, "VISA resource name out"=w632:refnum<visa-resource-name>)  [unwired: 6 in]
              }
            }
          }
          frame "set_fan" {
            # "Sets the fan speed."
            n201 = case shown="True" w640 {
              tunnel: w647 -> [_ w664]
              tunnel: w646 -> [w653 w662]
              tunnel: [w653 w661] -> w645
              tunnel: [w654 w660] -> w644
              tunnel: w643 -> [w654 w659]
              tunnel: w641 -> [w655 _]
              frame False {
                n202 = One Button Dialog(message=w655) -> ()  [unwired: 1 in, 1 out]
              }
              frame True {
                n203 = Unbundle By Name(w664) -> ("data"=w663:variant)
                n204 = Variant To Data(error in=w659, type=u8 0 ("Fan speed"), Variant=w663) -> (data=w656:u8, error out=w658:errorcluster)
                n205 = call <instrlib>:"Set fan speed.vi"("error in (no error)"=w658, "Fan speed"=w656, "VISA resource name"=w662) -> ("error out"=w660:errorcluster, "VISA resource name out"=w661:refnum<visa-resource-name>)  [unwired: 7 in]
              }
            }
          }
          frame "request_data" {
            # "This case is triggered by the timed loop. Another option would be to send a message to itself, but that causes a delay."
            n206 = case shown="True" w665 {
              tunnel: w680 -> [w684 w695]
              tunnel: [w684 w694] -> w679
              tunnel: [_ w693] -> w674
              tunnel: [_ w688] -> w670
              tunnel: w669 -> [w685 w687]
              tunnel: [w685 w686] -> w667
              tunnel: w666 -> [w683 _]
              frame False {
                n207 = One Button Dialog(message=w683) -> ()  [unwired: 1 in, 1 out]
                n208 = property on="Monitor data" class="Bool"("BoolText.Text"="Start" ("Boolean Text.Text")) -> ()  [unwired: 2 in, 2 out]
              }
              frame True {
                n209 = call <instrlib>:"Get Endstop Status.vi"("error in (no error)"=w687, "VISA resource name"=w695) -> ("error out"=w690:errorcluster, "End stop status"=w693:T12, "VISA resource name out"=w692:refnum<visa-resource-name>)  [unwired: 7 in]
                n210 = call <instrlib>:"Report temperatures.vi"("error in (no error)"=w690, "VISA resource name"=w692) -> ("error out"=w686:errorcluster, "Temperatures"=w691:T13, "VISA resource name out"=w694:refnum<visa-resource-name>)  [unwired: 7 in]
                n211 = Cluster To Array(cluster=w691) -> (array=w689:dbl[])
                n212 = Build Array(w689) -> (w688:dbl[][])
              }
            }
            "Temperature Chart" <- w670
            n213 = Unbundle(w674) -> ("x_min"=→"X min":bool, "y_min"=→"Y min":bool, "z_min"=→"Z min":bool)
          }
          frame "load_gcode" {
            # "The gcode file is loaded wron the selected path and is converted to an array of strings. This array is used to iterate through all gcodes."
            n214 = Select(t="Test mode", s="Test mode", f=w698) -> (s? t:f=w696:bool)
            n215 = case shown="True" w696 {
              tunnel: w707 -> [_ w724]
              tunnel: w706 -> [w712 w719]
              tunnel: [w712 w717] -> w702
              tunnel: [_ w716] -> w700
              tunnel: w699 -> [w711 _]
              frame False {
                n216 = One Button Dialog(message=w711) -> ()  [unwired: 1 in, 1 out]
                n217 = property on="Gcode file" class="Path"("Text.Text"="") -> ()  [unwired: 2 in, 2 out]
              }
              frame True {
                n218 = Unbundle By Name(w724) -> ("data"=w723:variant)
                n219 = Variant To Data(error in=w719, type=path "", Variant=w723) -> (data=w721:path, error out=w720:errorcluster)
                n220 = call "read Gcode.vi"("error in"=w720, "Gcode path (use dialog)"=w721) -> ("error out"=w715:errorcluster, "Gcode Array"=w716:string[])  [unwired: 7 in, 1 out]
                "Gcode array" <- w716
                n221 = property on="Gcode array" class="Arr (strict)"(error in=w715, "Index Values"=u32[] []) -> (error out=w714:errorcluster)  [unwired: 1 in, 1 out]
                n222 = property on="Start Gcode" class="Bool"(error in=w714, "DisabledEnum"=T3."Enabled" ("Disabled")) -> (error out=w717:errorcluster)  [unwired: 1 in, 1 out]
              }
            }
          }
          frame "run_gcode" {
            # "This case runs the indexed gcode from the gcode array. The index is increased by one every time this case is selected. The data is filetered and put in an XY graph because that's just awesome."
            n223 = Array Size(array=w746) -> (size(s)=w744:i32)
            n224 = Unbundle By Name(w756) -> ("data"=w757:variant)
            n225 = Variant To Data(error in=w755, type=0, Variant=w757) -> (data=w736:i32, error out=w752:errorcluster)
            n226 = Greater Or Equal?(x=w736, y=w744) -> (x >= y?=w743:bool)
            n227 = Increment(x=w736) -> (x+1=w735:i32)
            n228 = Index Array(array=w746, index=w736) -> (element=w738:string)
            n229 = call "build XY graph.vi"("Gcode line"=w738, "XY Graph in"=w739) -> ("XY Graph out"=w737:cluster{"X":dbl, "Y":dbl}[])  [unwired: 5 in]
            "XY Graph" <- w737
            n230 = property on="Test mode" class="Bool (strict)"() -> ("Value"=w725:bool)  [unwired: 2 in, 2 out]
            n231 = Subtract(x=w735, y=7) -> (x-y=w732:i32)
            n232 = case shown="True" w725 {
              tunnel: w753 -> [w764 w767]
              tunnel: w752 -> [w763 w766]
              tunnel: [w762 w767] -> w751
              tunnel: [w761 w766] -> _
              tunnel: w738 -> [w760 _]
              frame False {
                n233 = call <instrlib>:"Send raw Gcode.vi"("error in (no error)"=w763, "Gcode"=w760, "VISA resource name"=w764) -> ("error out"=w761:errorcluster, "VISA resource name out"=w762:refnum<visa-resource-name>)  [unwired: 5 in, 2 out]
              }
              frame True {
                n234 = Wait (ms)(milliseconds to wait=u32 5) -> ()  [unwired: 1 out]
              }
            }
            n235 = Less Or Equal To 0?(x=w732) -> (x <= 0?=w733:bool)
            n236 = Select(t=0, s=w733, f=w732) -> (s? t:f=w727:i32)
            n237 = Build Array(w727) -> (w726:i32[])
            n238 = property on="Gcode array" class="Arr (strict)"("Index Values"=w726) -> ()  [unwired: 2 in, 2 out]
            n239 = Increment(x=w736) -> (x+1=w745:i32)
            n240 = Select(t="finish_gcode" ("message"), s=w743, f="run_gcode" ("message")) -> (s? t:f=w740:string)
            n241 = Bundle(cluster=T4 {"message"="", "data"=variant} ("element"), "message"=w740, "data"=w745) -> (w749:T4)
            n242 = Enqueue Element(queue=w747, element=w749) -> (error out=w748:errorcluster)  [unwired: 2 in, 2 out]
          }
          frame "pause_gcode" {
            # "The pause gcode flushes the queue to prevent further messages from performing. The Z is raised by 5mm and the hotend can be moved with the manual controls if needed. If the pause button is selected again all flushed queue elements are put back into the queue and the gcode will run where it left off."
            n243 = Not(x=w777) -> (.not. x?=w775:bool)
            n244 = case shown="True" w775 {
              tunnel: w776 -> [w786 w797]
              tunnel: [w783 w796] -> w774
              tunnel: w773 -> [w783 _]
              tunnel: w772 -> [w785 w794]
              tunnel: [w784 w795] -> w771
              tunnel: w769 -> [w782 w793]
              tunnel: [w782 w792] -> w768
              frame False {
                n245 = for {
                  tunnel: w786 -> [w790]
                  tunnel: w783 -> [w789] mode=indexing
                  shift-right: [w787] -> w784
                  shift-left: w785 -> [w788]
                  n246 = Enqueue Element(queue=w790, element=w789, error in (no error)=w788) -> (error out=w787:errorcluster)  [unwired: 1 in, 2 out]
                }
              }
              frame True {
                n247 = property on="Test mode" class="Bool (strict)"() -> ("Value"=w791:bool)  [unwired: 2 in, 2 out]
                n248 = Flush Queue(queue=w797, error in (no error)=w794) -> (remaining elements=w796:T4[], error out=w795:errorcluster)  [unwired: 1 out]
                n249 = case shown="False" w791 {
                  tunnel: w793 -> [w807 w809]
                  tunnel: [w799 w809] -> w792
                  frame False {
                    n250 = call <instrlib>:"Positioning.vi"("type"=enum16{"Absolute (G90)", "Relative (G91)"}."Relative (G91)", "VISA resource name"=w807) -> ("error out"=w805:errorcluster, "VISA resource name out"=w808:refnum<visa-resource-name>)  [unwired: 8 in]
                    n251 = Bundle By Name(cluster=T10 {"E"=0.0, "F"=0.0, "X"=0.0, "Y"=0.0, "Z"=0.0} ("Distances"), "Z"=5.0) -> (w800:T10)
                    n252 = call <instrlib>:"Move.vi"("error in (no error)"=w805, "Distances"=w800, "VISA resource name"=w808) -> ("error out"=w804:errorcluster, "VISA resource name out"=w803:refnum<visa-resource-name>)  [unwired: 7 in]
                    n253 = call <instrlib>:"Positioning.vi"("error in (no error)"=w804, "type"=enum16{"Absolute (G90)", "Relative (G91)"}."Absolute (G90)", "VISA resource name"=w803) -> ("VISA resource name out"=w799:refnum<visa-resource-name>)  [unwired: 7 in, 1 out]
                  }
                  frame True {
                  }
                }
              }
            }
          }
          frame "stop_gcode" {
            (unwired) 0 ("Top Row")
            (unwired) string[] [] ("Item Names")
            w813 = T3."Disabled and Grayed Out" ("Disabled")
            # "The gcode is stopped and the queue is flushed and forgotten to prevent further actions."
            n254 = Flush Queue(queue=w817, error in (no error)=w816) -> (error out=w815:errorcluster)  [unwired: 2 out]
            n255 = invoke on="XY Graph" class="XYGraph (strict)" method="Reinit To Default"() -> ()  [unwired: 3 in, 3 out]
            n256 = invoke on="Gcode file" class="Path" method="Reinit To Default"() -> ()  [unwired: 3 in, 3 out]
            n257 = property on="Gcode array" class="Arr (strict)"("Index Values"=u32[] [], "Val(Sgnl)"=string[] [] ("Value (Signaling)")) -> ()  [unwired: 2 in, 2 out]
            n258 = property on="Pause Gcode" class="Bool"("DisabledEnum"=w813) -> ()  [unwired: 2 in, 2 out]
            n259 = property on="Stop Gcode" class="Bool"("DisabledEnum"=w813) -> ()  [unwired: 2 in, 2 out]
            n260 = property on="Start Gcode" class="Bool"("DisabledEnum"=w813) -> ()  [unwired: 2 in, 2 out]
          }
          frame "finish_gcode" {
            (unwired) string[] [] ("Item Names")
            w825 = T3."Disabled and Grayed Out" ("Disabled")
            # "The gcode is stopped but on a positive note."
            n261 = invoke on="XY Graph" class="XYGraph (strict)" method="Reinit To Default"() -> ()  [unwired: 3 in, 3 out]
            n262 = invoke on="Gcode file" class="Path" method="Reinit To Default"() -> ()  [unwired: 3 in, 3 out]
            n263 = property on="Gcode array" class="Arr (strict)"("Index Values"=u32[] [], "Val(Sgnl)"=string[] [] ("Value (Signaling)")) -> ()  [unwired: 2 in, 2 out]
            n264 = One Button Dialog(message="Gcode finished!") -> ()  [unwired: 1 in, 1 out]
            n265 = property on="Pause Gcode" class="Bool"("DisabledEnum"=w825) -> ()  [unwired: 2 in, 2 out]
            n266 = property on="Stop Gcode" class="Bool"("DisabledEnum"=w825) -> ()  [unwired: 2 in, 2 out]
            n267 = property on="Start Gcode" class="Bool"("DisabledEnum"=w825) -> ()  [unwired: 2 in, 2 out]
          }
          frame "start_torture" {
            # "The torture sequence is started. The printer is homed after which the head is placed into the center at a Z height of 10mm. The torture sequence is selected."
            n268 = Select(t="Test mode", s="Test mode", f=w836) -> (s? t:f=w837:bool)
            n269 = case shown="True" w837 {
              tunnel: w845 -> [w854 w863]
              tunnel: w844 -> [w853 w862]
              tunnel: "Axle" -> [_ w861]
              tunnel: w841 -> [_ w860]
              tunnel: [w853 w858] -> w840
              tunnel: [w854 w856] -> w839
              tunnel: "Test mode" -> [_ w855]
              tunnel: w835 -> [w852 _]
              frame False {
                n270 = One Button Dialog(message=w852) -> ()  [unwired: 1 in, 1 out]
                n271 = property on="Start torture" class="Bool"("BoolText.Text"="Start" ("Boolean Text.Text")) -> ()  [unwired: 2 in, 2 out]
              }
              frame True {
                n272 = case shown="False" w855 {
                  tunnel: w863 -> [w875 w896]
                  tunnel: w862 -> [w874 w897]
                  tunnel: w861 -> [w871 _]
                  tunnel: [w865 w897] -> w857
                  tunnel: [w864 w896] -> w856
                  frame False {
                    n273 = property on="Distance" class="Slide (strict)"() -> ("Value"=w872:dbl)  [unwired: 2 in, 2 out]
                    n274 = property on="X" class="DigNum (strict)"() -> ("Value"=w884:dbl)  [unwired: 2 in, 2 out]
                    n275 = property on="Y" class="DigNum (strict)"() -> ("Value"=w881:dbl)  [unwired: 2 in, 2 out]
                    n276 = Divide(x=w884, y=2.0) -> (x/y=w869:dbl)
                    n277 = Divide(x=w881, y=2.0) -> (x/y=w867:dbl)
                    n278 = Divide(x=w872, y=2.0) -> (x/y=w866:dbl)
                    n279 = case shown="\"Y\"" w871 {
                      tunnel: [w889 w895] -> w870
                      tunnel: w869 -> [w890 w895]
                      tunnel: w866 -> [w891 _]
                      tunnel: [w888 w892] -> w868
                      tunnel: w867 -> [w888 w893]
                      tunnel: w866 -> [_ w894]
                      frame "X", Default {
                        n280 = Subtract(x=w890, y=w891) -> (x-y=w889:dbl)
                      }
                      frame "Y" {
                        n281 = Subtract(x=w893, y=w894) -> (x-y=w892:dbl)
                      }
                    }
                    n282 = call <instrlib>:"Home.vi"("error in (no error)"=w874, "VISA resource name"=w875) -> ("error out"=w877:errorcluster, "VISA resource name out"=w876:refnum<visa-resource-name>)  [unwired: 8 in]
                    n283 = call <instrlib>:"Positioning.vi"("error in (no error)"=w877, "type"=enum16{"Absolute (G90)", "Relative (G91)"}."Absolute (G90)", "VISA resource name"=w876) -> ("error out"=w886:errorcluster, "VISA resource name out"=w887:refnum<visa-resource-name>)  [unwired: 7 in]
                    n284 = Bundle By Name(cluster=T10 {"E"=0.0, "F"=0.0, "X"=0.0, "Y"=0.0, "Z"=0.0} ("Distances"), "X"=w870, "Y"=w868, "Z"=10.0) -> (w878:T10)
                    n285 = call <instrlib>:"Move.vi"("error in (no error)"=w886, "Distances"=w878, "VISA resource name"=w887) -> ("error out"=w865:errorcluster, "VISA resource name out"=w864:refnum<visa-resource-name>)  [unwired: 7 in]
                  }
                  frame True {
                  }
                }
                n286 = Enqueue Element(queue=w860, element=T4 {"message"="torture", "data"=variant}, error in (no error)=w857) -> (error out=w858:errorcluster)  [unwired: 1 in, 2 out]
              }
            }
          }
          frame "torture" {
            # "This sequence moves the print head symmetric from the bed center back and forth without waiting. The frequence can be changed by changing the travel distance or movement speed. This case calls itself to stay in a loop."
            n287 = Divide(x="Distance", y=2.0) -> (x/y=w907:dbl)
            n288 = property on="Axle" class="Enum (strict)"() -> ("Value"=w910:enum16{"X", "Y", "Z"})  [unwired: 2 in, 2 out]
            n289 = case shown="\"Y\"" w910 {
              tunnel: T10 {"E"=0.0, "F"=0.0, "X"=0.0, "Y"=0.0, "Z"=0.0} ("Distances") -> [w945 w955]
              tunnel: [w944 w956] -> w919
              tunnel: "Speed" -> [w943 w954]
              tunnel: w907 -> [w937 w948]
              tunnel: w906 -> [w939 w950]
              tunnel: [w936 w947] -> w898
              tunnel: [w935 w946] -> w902
              frame "X", Default {
                n290 = property on="X" class="DigNum (strict)"() -> ("Value"=w936:dbl)  [unwired: 2 in, 2 out]
                n291 = Divide(x=w936, y=2.0) -> (x/y=w938:dbl)
                n292 = Add(x=w938, y=w937) -> (x+y=w941:dbl)
                n293 = Subtract(x=w938, y=w937) -> (x-y=w940:dbl)
                n294 = Select(t=w941, s=w939, f=w940) -> (s? t:f=w935:dbl)
                n295 = Bundle By Name(cluster=w945, "F"=w943, "X"=w935) -> (w944:T10)
              }
              frame "Y" {
                n296 = property on="Y" class="DigNum (strict)"() -> ("Value"=w947:dbl)  [unwired: 2 in, 2 out]
                n297 = Divide(x=w947, y=2.0) -> (x/y=w949:dbl)
                n298 = Add(x=w949, y=w948) -> (x+y=w952:dbl)
                n299 = Subtract(x=w949, y=w948) -> (x-y=w951:dbl)
                n300 = Select(t=w952, s=w950, f=w951) -> (s? t:f=w946:dbl)
                n301 = Bundle By Name(cluster=w955, "F"=w954, "Y"=w946) -> (w956:T10)
              }
            }
            "Position sent" <- w902
            n302 = Not(x=w906) -> (.not. x?=w905:bool)
            n303 = property on="Test mode" class="Bool (strict)"() -> ("Value"=w904:bool)  [unwired: 2 in, 2 out]
            n304 = Equal To 0?(x=w898) -> (x = 0?=w901:bool)
            n305 = case shown="True" w904 {
              tunnel: w919 -> [w931 _]
              tunnel: w918 -> [w930 w933]
              tunnel: w917 -> [w929 w932]
              tunnel: [w928 w932] -> w916
              tunnel: [w927 w933] -> w914
              frame False {
                n306 = call <instrlib>:"Move.vi"("error in (no error)"=w930, "Distances"=w931, "VISA resource name"=w929) -> ("error out"=w927:errorcluster, "VISA resource name out"=w928:refnum<visa-resource-name>)  [unwired: 7 in]
              }
              frame True {
                n307 = Wait (ms)(milliseconds to wait=u32 200) -> ()  [unwired: 1 out]
              }
            }
            n308 = Select(t=300.0, s=w901, f=w898) -> (s? t:f=w900:dbl)
            n309 = property on="Distance" class="Slide (strict)"("Scale.Minimum"=0.0 ("Scale.Range:Minimum"), "Scale.Maximum"=w900) -> ()  [unwired: 2 in, 2 out]
            n310 = Enqueue Element(queue=w912, element=T4 {"message"="torture", "data"=variant}, error in (no error)=w914) -> (error out=w913:errorcluster)  [unwired: 1 in, 2 out]
          }
          frame "stop_torture" {
            # "The queue is flushed so the remaining torture messages aren't performed anymore."
            n311 = Flush Queue(queue=w959, error in (no error)=w958) -> (error out=w957:errorcluster)  [unwired: 2 out]
          }
          frame "close" {
            # "This closes the port and ends the loop."
          }
        }
      }
      frame Error {
        # "This case is selected when the Dequeue element generates an error. This means that the queue is released and this loop is stopped."
      }
    }
    n312 = call <vilib>:"Clear Errors.vi"("error in (no error)"=w335, "specific error code to clear (0: all)"=1) -> ("error out"=w334:errorcluster)  [unwired: 4 in, 1 out]
    n313 = call <vilib>:"Simple Error Handler.vi"("error in (no error)"=w334) -> ("error out"=w328:errorcluster)  [unwired: 4 in, 4 out]
  }
  n314 = node-c288(w28) -> ()  [unwired: 1 out]
  n315 = Release Queue(queue=w9, error in (no error)=w44) -> ()  [unwired: 1 in, 3 out]
  n316 = call <instrlib>:"Close.vi"("VISA resource name"=w8) -> ("error out"=w7:errorcluster)  [unwired: 10 in]
  n317 = call <vilib>:"Close Config Data.vi"("refnum"=w35) -> ("error out"=w6:errorcluster)  [unwired: 9 in, 1 out]
  n318 = call <vilib>:"Clear Errors.vi"("error in (no error)"=w7) -> ()  [unwired: 5 in, 2 out]
  n319 = call <vilib>:"Clear Errors.vi"("error in (no error)"=w6) -> ("error out"=w5:errorcluster)  [unwired: 5 in, 1 out]
  n320 = property class="VI"(error in=w5, "Front Panel Window:Open"=FALSE) -> ()  [unwired: 1 in, 2 out]
